vi "calibrate XYZ positions.vi"   [LabVIEW 2012]
doc: "SciScan 1.2 160622"
uses:
  GFG/GFGnumericGet.vi
  GFG/GFGstringGet.vi
  GFG/GFG library.lvlib
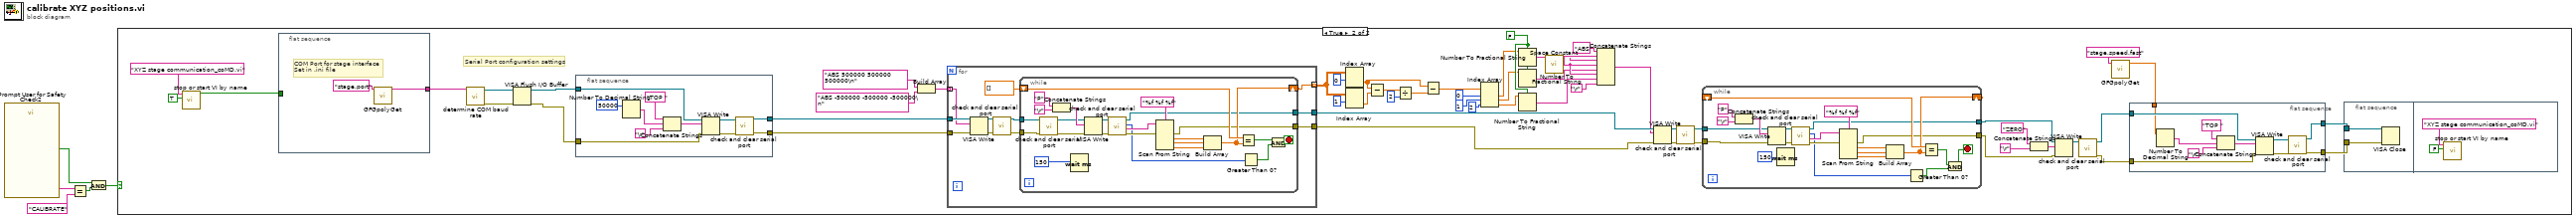
[diagram p0: block diagram]
diagram:
  n1 = call "Prompt User for Safety Check2"() -> ("Type here:"=w2:string, "OK"=w4:bool)  [unwired: 17 in, 1 out]
  n2 = Equal?(x=w2, y="CALIBRATE") -> (x = y?=w5:bool)
  n3 = And(x=w4, y=w5) -> (x .and. y?=w1:bool)
  n4 = case shown="True" w1 {
    frame False {
    }
    frame True {
      w35 = FALSE ("use system decimal point (T)")
      # "Serial Port configuration settings"
      n5 = call "stop or start VI by name.vi"("stop (T) or start (F)"=TRUE, "VI name"="XYZ stage communication_coMD.vi") -> ("VI is running"=w53:bool)  [unwired: 9 in]
      n6 = flat-sequence {
        tunnel: [w132] -> w59
        tunnel: w53 -> [_]
        frame #0 {
          # "COM Port for stage interface\nSet in .ini file"
          n7 = call-poly "GFGpolyGet.vi"("Variable Name in"="stage.port") -> ("String"=w132:string)  [unwired: 9 in, 1 out]
        }
      }
      n8 = call "determine COM baud rate.vi"("VISA resource name"=w59) -> ("error out"=w57:errorcluster, "VISA resource name out"=w58:refnum<visa-resource-name>)  [unwired: 8 in, 1 out]
      n9 = VISA Flush I/O Buffer(VISA resource name=w58, error in (no error)=w57) -> (VISA resource name out=w56:refnum<visa-resource-name>, error out=w55:errorcluster)  [unwired: 1 in]
      n10 = flat-sequence {
        tunnel: w56 -> [w138]
        tunnel: w55 -> [w137]
        tunnel: [w135] -> w47
        tunnel: [w134] -> w48
        frame #0 {
          n11 = Number To Decimal String(number=50000) -> (decimal integer string=w144:string)  [unwired: 1 in]
          n12 = Concatenate Strings("TOP " ("write buffer"), w144, "\r") -> (w141:string)
          n13 = VISA Write(VISA resource name=w138, write buffer=w141, error in (no error)=w137) -> (VISA resource name out=w140:refnum<visa-resource-name>, error out=w136:errorcluster)  [unwired: 1 out]
          n14 = call "check and clear serial port.vi"("error in (no error)"=w136, "VISA resource name in"=w140) -> ("error out"=w135:errorcluster, "VISA resource name out"=w134:refnum<visa-resource-name>)  [unwired: 6 in, 2 out]
        }
      }
      n15 = Build Array("ABS 500000 500000 500000\n" ("write buffer"), "ABS -500000 -500000 -500000\n" ("write buffer")) -> (w44:string[])
      n16 = for {
        tunnel: w48 -> [w91]
        tunnel: w47 -> [w90]
        tunnel: [w86] -> w21
        tunnel: [w85] -> w20
        tunnel: w44 -> [w84] mode=indexing
        tunnel: [w83] -> w43 mode=indexing
        n17 = VISA Write(VISA resource name=w91, write buffer=w84, error in (no error)=w90) -> (VISA resource name out=w92:refnum<visa-resource-name>, error out=w89:errorcluster)  [unwired: 1 out]
        n18 = call "check and clear serial port.vi"("error in (no error)"=w89, "VISA resource name in"=w92) -> ("error out"=w87:errorcluster, "VISA resource name out"=w88:refnum<visa-resource-name>)  [unwired: 6 in, 2 out]
        n19 = while {
          shift-right: [w104] -> w83
          shift-left: dbl[] [] -> [w105]
          tunnel: w88 -> [w99]
          tunnel: w87 -> [w101]
          tunnel: [w103] -> w86
          tunnel: [w102] -> w85
          stop <- w97 stop-if-true
          n20 = call "check and clear serial port.vi"("error in (no error)"=w101, "VISA resource name in"=w99) -> ("error out"=w100:errorcluster, "VISA resource name out"=w98:refnum<visa-resource-name>)  [unwired: 6 in, 2 out]
          n21 = Concatenate Strings("P" ("write buffer"), "\r") -> (w113:string)
          n22 = Wait (ms)(milliseconds to wait=u32 150) -> ()  [unwired: 1 out]
          n23 = VISA Write(VISA resource name=w98, write buffer=w113, error in (no error)=w100) -> (VISA resource name out=w110:refnum<visa-resource-name>, error out=w109:errorcluster)  [unwired: 1 out]
          n24 = call "check and clear serial port.vi"("error in (no error)"=w109, "VISA resource name in"=w110) -> ("error out"=w111:errorcluster, "read buffer"=w112:string, "number of bytes actually read"=w95:u32, "VISA resource name out"=w103:refnum<visa-resource-name>)  [unwired: 6 in]
          n25 = Scan From String(format string="%f %f %f", input string=w112, error in=w111) -> (error out=w102:errorcluster, output 1=w116:dbl, output 2=w115:dbl, output 3=w114:dbl)  [unwired: 4 in, 2 out]
          n26 = Build Array(w116, w115, w114) -> (w104:dbl[])
          n27 = Equal?(x=w105, y=w104) -> (x = y?=w93:bool)
          n28 = Greater Than 0?(x=w95) -> (x > 0?=w96:bool)
          n29 = And(x=w93, y=w96) -> (x .and. y?=w97:bool)
        }
      }
      n30 = Index Array(array=w43, index (row)=0) -> (element=w36:dbl[])  [unwired: 1 in]
      n31 = Index Array(array=w43, index (row)=1) -> (element=w40:dbl[])  [unwired: 1 in]
      n32 = Subtract(x=w36, y=w40) -> (x-y=w39:dbl[])
      n33 = Divide(x=w39, y=2) -> (x/y=w37:dbl[])
      n34 = Subtract(x=w36, y=w37) -> (x-y=w28:dbl[])
      n35 = Index Array(array=w28, index #1=0 ("index"), index #2=1 ("index"), index #3=2 ("index")) -> (element #1=w24:dbl, element #2=w23:dbl, element #3=w22:dbl)
      n36 = Number To Fractional String(use system decimal point (T)=w35, number=w24) -> (F-format string=w29:string)  [unwired: 2 in]
      n37 = Number To Fractional String(use system decimal point (T)=w35, number=w23) -> (F-format string=w30:string)  [unwired: 2 in]
      n38 = Number To Fractional String(use system decimal point (T)=w35, number=w22) -> (F-format string=w31:string)  [unwired: 2 in]
      n39 = call <vilib>:"Space Constant.vi"() -> ("String"=w32:string)
      n40 = Concatenate Strings("ABS" ("string"), w32, w29, w32, w30, w32, w31, "\r") -> (w15:string)
      n41 = VISA Write(VISA resource name=w21, write buffer=w15, error in (no error)=w20) -> (VISA resource name out=w19:refnum<visa-resource-name>, error out=w18:errorcluster)  [unwired: 1 out]
      n42 = call "check and clear serial port.vi"("error in (no error)"=w18, "VISA resource name in"=w19) -> ("error out"=w16:errorcluster, "VISA resource name out"=w17:refnum<visa-resource-name>)  [unwired: 6 in, 2 out]
      n43 = while {
        shift-right: [w69] -> _
        shift-left: _ -> [w70]
        tunnel: w17 -> [w68]
        tunnel: w16 -> [w67]
        tunnel: [w66] -> w10
        tunnel: [w65] -> w9
        stop <- w62 stop-if-true
        n44 = Concatenate Strings("P" ("write buffer"), "\r") -> (w78:string)
        n45 = VISA Write(VISA resource name=w68, write buffer=w78, error in (no error)=w67) -> (VISA resource name out=w75:refnum<visa-resource-name>, error out=w74:errorcluster)  [unwired: 1 out]
        n46 = Wait (ms)(milliseconds to wait=u32 150) -> ()  [unwired: 1 out]
        n47 = call "check and clear serial port.vi"("error in (no error)"=w74, "VISA resource name in"=w75) -> ("error out"=w76:errorcluster, "read buffer"=w77:string, "number of bytes actually read"=w60:u32, "VISA resource name out"=w66:refnum<visa-resource-name>)  [unwired: 6 in]
        n48 = Scan From String(format string="%f %f %f", input string=w77, error in=w76) -> (error out=w65:errorcluster, output 1=w81:dbl, output 2=w80:dbl, output 3=w79:dbl)  [unwired: 4 in, 2 out]
        n49 = Build Array(w81, w80, w79) -> (w69:dbl[])
        n50 = Greater Than 0?(x=w60) -> (x > 0?=w61:bool)
        n51 = Equal?(x=w70, y=w69) -> (x = y?=w63:bool)
        n52 = And(x=w63, y=w61) -> (x .and. y?=w62:bool)
      }
      n53 = Concatenate Strings("ZERO" ("write buffer"), "\r") -> (w14:string)
      n54 = VISA Write(VISA resource name=w10, write buffer=w14, error in (no error)=w9) -> (VISA resource name out=w13:refnum<visa-resource-name>)  [unwired: 2 out]
      n55 = call "check and clear serial port.vi"("VISA resource name in"=w13) -> ("error out"=w8:errorcluster, "VISA resource name out"=w7:refnum<visa-resource-name>)  [unwired: 7 in, 2 out]
      n56 = call-poly "GFGpolyGet.vi"("Variable Name in"="stage.speed.fast") -> ("Numeric"=w49:dbl)  [unwired: 8 in, 2 out]
      n57 = flat-sequence {
        tunnel: w7 -> [w126]
        tunnel: w8 -> [w125]
        tunnel: [w123] -> w52
        tunnel: [w122] -> w51
        tunnel: w49 -> [w121]
        frame #0 {
          n58 = Number To Decimal String(number=w121) -> (decimal integer string=w131:string)  [unwired: 1 in]
          n59 = Concatenate Strings("TOP " ("write buffer"), w131, "\r") -> (w128:string)
          n60 = VISA Write(VISA resource name=w126, write buffer=w128, error in (no error)=w125) -> (VISA resource name out=w127:refnum<visa-resource-name>, error out=w124:errorcluster)  [unwired: 1 out]
          n61 = call "check and clear serial port.vi"("error in (no error)"=w124, "VISA resource name in"=w127) -> ("error out"=w123:errorcluster, "VISA resource name out"=w122:refnum<visa-resource-name>)  [unwired: 6 in, 2 out]
        }
      }
      n62 = flat-sequence {
        tunnel: w52 -> [w118]
        tunnel: w51 -> [w117]
        frame #0 {
          n63 = VISA Close(VISA resource name=w117, error in (no error)=w118) -> ()  [unwired: 1 out]
        }
        frame #1 {
          n64 = call "stop or start VI by name.vi"("stop (T) or start (F)"=FALSE, "VI name"="XYZ stage communication_coMD.vi") -> ()  [unwired: 9 in, 1 out]
        }
      }
    }
  }
